vi "6a.vi"() -> ()   [LabVIEW 2015]
panel:
  out "Signals":dbl[][](graph)
  in  "# of record":i32=20
  out "Data record":i32
  in  "physical channels":tag="Dev1/ai0:2"
  in  "Sampling rate":dbl=10000.0
  in  "# of samples":i32=500
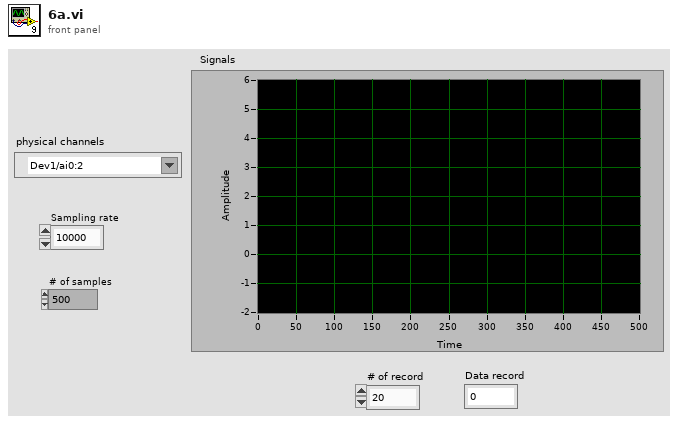
[diagram p1: front panel]
types:
  T1 = enum16{"open", "replace", "create", "open or create", "replace or create", "replace or create with confirmation"}
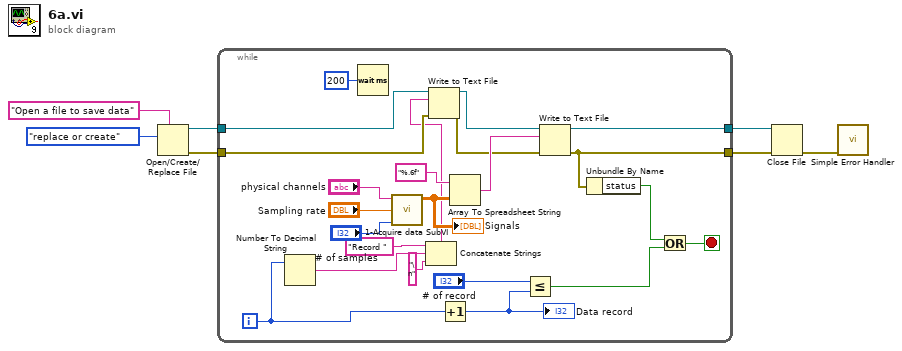
[diagram p0: block diagram]
diagram:
  n1 = Open/Create/Replace File(prompt="Open a file to save data", operation (0:open)=T1."replace or create") -> (refnum out=w7:refnum<file>, error out=w5:errorcluster)  [unwired: 4 in, 1 out]
  n2 = while {
    tunnel: w7 -> [w16]
    tunnel: [w30] -> w6
    tunnel: w5 -> [w15]
    tunnel: [w27] -> w4
    i -> [w12]
    stop <- w25 stop-if-true
    n3 = Number To Decimal String(number=w12) -> (decimal integer string=w10:string)  [unwired: 1 in]
    n4 = Wait (ms)(milliseconds to wait=u32 200) -> ()  [unwired: 1 out]
    n5 = call "1-Acquire data SubVI.vi"("# of samples/channel"="# of samples", "Sampling rate"="Sampling rate", "physical channels"="physical channels") -> ("data"=w17:dbl[][])  [unwired: 8 in]
    "Signals" <- w17
    n6 = Concatenate Strings("Record " ("string"), w10, "\n" ("string")) -> (w9:string)
    n7 = Write to Text File(file (use dialog)=w16, text=w9, error in=w15) -> (refnum out=w14:refnum<file>, error out=w13:errorcluster)  [unwired: 1 in, 1 out]
    n8 = Increment(x=w12) -> (x+1=w22:i32)
    "Data record" <- w22
    n9 = Array To Spreadsheet String(array=w17, 3:"%.6f" ("format string")) -> (spreadsheet string=w28:string)  [unwired: 1 in]
    n10 = Less Or Equal?(x="# of record", y=w22) -> (x <= y?=w21:bool)
    n11 = Write to Text File(file (use dialog)=w14, text=w28, error in=w13) -> (refnum out=w30:refnum<file>, error out=w27:errorcluster)  [unwired: 1 in, 1 out]
    n12 = Unbundle By Name(w27) -> ("status"=w26:bool)
    n13 = Or(x=w26, y=w21) -> (x .or. y?=w25:bool)
  }
  n14 = Close File(refnum=w6, error in=w4) -> (error out=w1:errorcluster)  [unwired: 1 out]
  n15 = call <vilib>:"Simple Error Handler.vi"("error in (no error)"=w1) -> ()  [unwired: 4 in, 5 out]
